vi "11_ПростейшийВП_Expression Node.vi"() -> ()   [LabVIEW 2016]
panel:
  out "Y":dbl
  in  "X":dbl
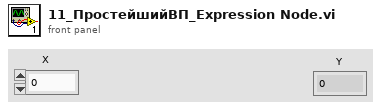
[diagram p1: front panel]
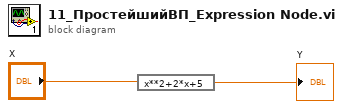
[diagram p0: block diagram]
diagram:
  n1 = expression code="x**2+2*x+5"("X") -> (→"Y":dbl)
